vi "DataBuffer_NET-2.vi"() -> ()   [LabVIEW 2016]
uses:
  C:/Program Files/Ocean Optics/OmniDriver/OOI_HOME/NETOmniDriver-NET20.dll
  Program Files/Ocean Optics/OmniDriver/OOI_HOME/NETOmniDriver-NET20.dll
panel:
  out "isFeatureSupportedDataBuffer":i16
  out "getBufferCapacity":i32
  in  "param0":i32
  in  "spectrometerIndex":i32
  out "Spectrometer Name:":string
  out "Serial Number:":string
  in  "Scans to Average":i32=1 min=1 max=50 step=1
  in  "Boxcar Width":i32=5 min=0 max=50 step=1
  in  "Int. Time (microsec)":i32=100000 min=3000 max=65000000
  out "Number of Spectrometers":i32
  in  "stop":bool
  out "Current Spectrum":cluster{"Y":dbl[], "Y":dbl[]}[](graph)
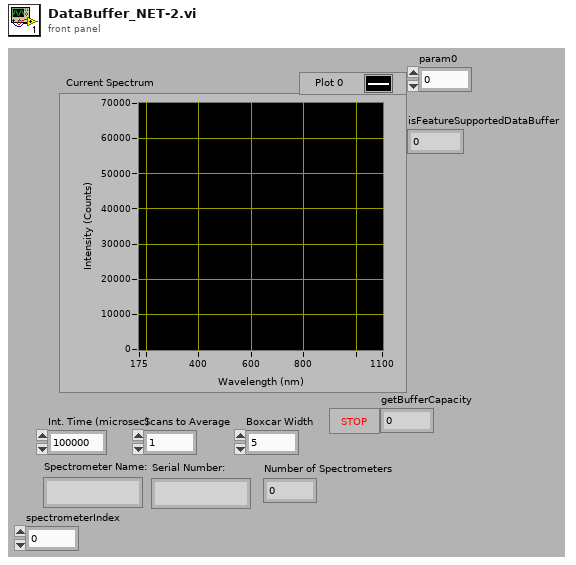
[diagram p1: front panel]
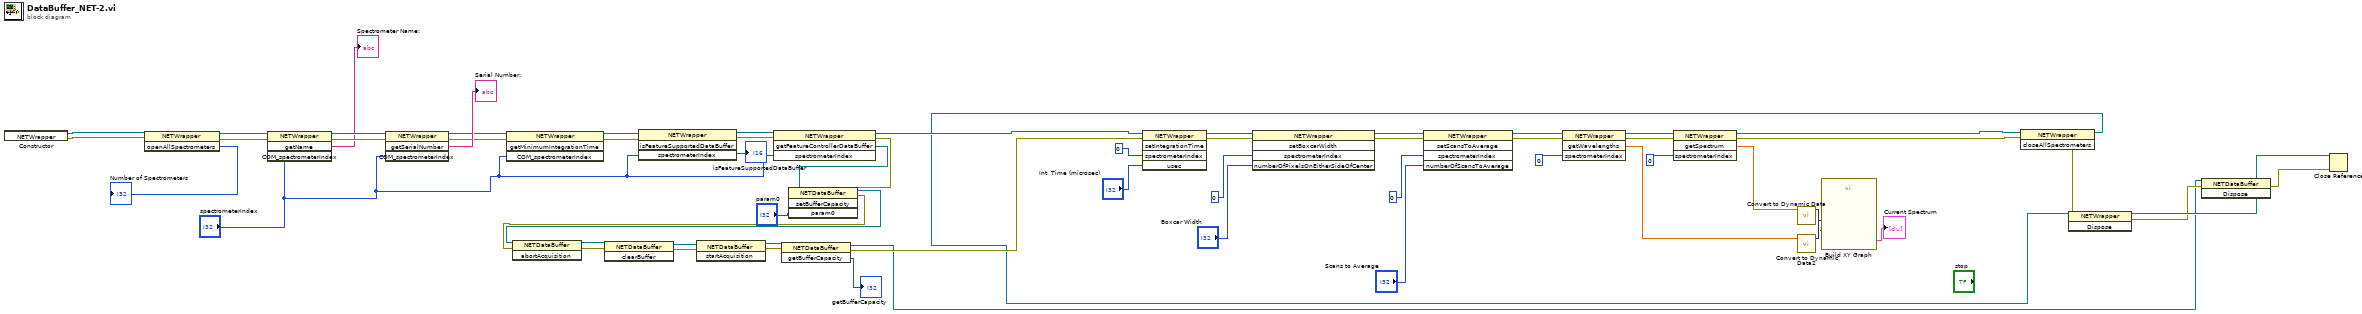
[diagram p0: block diagram]
diagram:
  n1 = constructor class="NETWrapper"() -> (reference out=w47:refnum<k24>, error out=w46:errorcluster)  [unwired: 3 in, 1 out]
  n2 = invoke class="NETWrapper" method="openAllSpectrometers"(reference=w47, error in=w46) -> (reference out=w56:refnum<k24>, error out=w55:errorcluster, "openAllSpectrometers"=→"Number of Spectrometers":i32)  [unwired: 1 in]
  n3 = invoke class="NETWrapper" method="getName"(reference=w56, error in=w55, "COM_spectrometerIndex"="spectrometerIndex") -> (reference out=w54:refnum<k24>, error out=w53:errorcluster, "getName"=→"Spectrometer Name:":string)  [unwired: 1 in, 1 out]
  n4 = invoke class="NETWrapper" method="getSerialNumber"(reference=w54, error in=w53, "COM_spectrometerIndex"="spectrometerIndex") -> (reference out=w51:refnum<k24>, error out=w50:errorcluster, "getSerialNumber"=→"Serial Number:":string)  [unwired: 1 in, 1 out]
  n5 = invoke class="NETWrapper" method="getMinimumIntegrationTime"(reference=w51, error in=w50, "COM_spectrometerIndex"="spectrometerIndex") -> (reference out=w45:refnum<k24>, error out=w44:errorcluster)  [unwired: 1 in, 2 out]
  n6 = invoke class="NETWrapper" method="isFeatureSupportedDataBuffer"(reference=w45, error in=w44, "spectrometerIndex"="spectrometerIndex") -> (reference out=w43:refnum<k24>, error out=w42:errorcluster, "isFeatureSupportedDataBuffer"=→"isFeatureSupportedDataBuffer":i16)  [unwired: 1 in, 1 out]
  n7 = invoke class="NETWrapper" method="getFeatureControllerDataBuffer"(reference=w43, error in=w42, "spectrometerIndex"="spectrometerIndex") -> (reference out=w41:refnum<k24>, error out=w33:errorcluster, "getFeatureControllerDataBuffer"=w35:refnum<k24>)  [unwired: 1 in, 1 out]
  n8 = invoke class="NETDataBuffer" method="setBufferCapacity"(reference=w35, error in=w33, "param0"="param0") -> (reference out=w34:refnum<k24>, error out=w31:errorcluster)  [unwired: 1 in, 2 out]
  n9 = invoke class="NETDataBuffer" method="abortAcquisition"(reference=w34, error in=w31) -> (reference out=w39:refnum<k24>, error out=w38:errorcluster)  [unwired: 1 in, 1 out]
  n10 = invoke class="NETDataBuffer" method="clearBuffer"(reference=w39, error in=w38) -> (reference out=w37:refnum<k24>, error out=w36:errorcluster)  [unwired: 1 in, 1 out]
  n11 = invoke class="NETDataBuffer" method="startAcquisition"(reference=w37, error in=w36) -> (reference out=w28:refnum<k24>, error out=w27:errorcluster)  [unwired: 1 in, 1 out]
  n12 = invoke class="NETDataBuffer" method="getBufferCapacity"(reference=w28, error in=w27) -> (reference out=w22:refnum<k24>, error out=w32:errorcluster, "getBufferCapacity"=→"getBufferCapacity":i32)  [unwired: 1 in]
  n13 = invoke class="NETWrapper" method="setIntegrationTime"(reference=w41, error in=w32, "spectrometerIndex"=0, "usec"="Int. Time (microsec)") -> (reference out=w11:refnum<k24>, error out=w10:errorcluster)  [unwired: 1 in, 3 out]
  n14 = invoke class="NETWrapper" method="setBoxcarWidth"(reference=w11, error in=w10, "spectrometerIndex"=0, "numberOfPixelsOnEitherSideOfCenter"="Boxcar Width") -> (reference out=w8:refnum<k24>, error out=w7:errorcluster)  [unwired: 1 in, 3 out]
  n15 = invoke class="NETWrapper" method="setScansToAverage"(reference=w8, error in=w7, "spectrometerIndex"=0, "numberOfScansToAverage"="Scans to Average") -> (reference out=w4:refnum<k24>, error out=w3:errorcluster)  [unwired: 1 in, 3 out]
  n16 = invoke class="NETWrapper" method="getWavelengths"(reference=w4, error in=w3, "spectrometerIndex"=0) -> (reference out=w20:refnum<k24>, error out=w19:errorcluster, "getWavelengths"=w1:dbl[])  [unwired: 1 in, 1 out]
  n17 = invoke class="NETWrapper" method="getSpectrum"(reference=w20, error in=w19, "spectrometerIndex"=0) -> (reference out=w59:refnum<k24>, error out=w60:errorcluster, "getSpectrum"=w2:dbl[])  [unwired: 1 in, 1 out]
  n18 = call "Convert to Dynamic Data"("Array"=w2) -> ("Dynamic Data Type"=w16:dynamicdata)  [unwired: 3 out]
  n19 = call "Convert to Dynamic Data2"("Array"=w1) -> ("Dynamic Data Type"=w17:dynamicdata)  [unwired: 3 out]
  n20 = call "Build XY Graph"("Y Input"=w16, "X Input"=w17) -> ("XY Graph"=→"Current Spectrum":cluster{"Y":dbl[], "Y":dbl[]}[])  [unwired: 3 in, 6 out]
  n21 = invoke class="NETWrapper" method="closeAllSpectrometers"(reference=w59, error in=w60) -> (reference out=w23:refnum<k24>, error out=w49:errorcluster)  [unwired: 1 in, 1 out]
  n22 = invoke class="NETWrapper" method="Dispose"(reference=w23, error in=w49) -> (reference out=w48:refnum<k24>, error out=w25:errorcluster)  [unwired: 1 in, 1 out]
  n23 = invoke class="NETDataBuffer" method="Dispose"(reference=w22, error in=w25) -> (error out=w24:errorcluster)  [unwired: 1 in, 2 out]
  n24 = Close Reference(reference=w48, error in (no error)=w24) -> ()  [unwired: 1 out]
